vi "_BMarkInfo to MCTable.vi"(11 "BookmarkInfo":T1=[{"Bookmark ID"=1689, "Bookmark Tag"="#CSM", "Label Text"="#CSM State Syntax\n\n// Comment line, all text to the right of “//” will be ignored\n// Local Message Example\nDoSth: DoA >> Arguments\n\n// Sync Call Example\nAPI: xxxx >> Arguments -@ TargetModule\n\n// Async Call Example\nAPI: xxxx >> Arguments -> TargetModule\n\n// Async Call without Reply Example\nAPI: xxxx >> Arguments ->| TargetModule\n\n// Broadcast normal status:\nStatus >> StatusArguments  -><status>\n\n// Broadcast Interrupt status:\nInterrupt >> StatusArguments  -><interrupt>\n\n// Register Source Module's status to Handler Module\nStatus@Source Module >> Handler Module@Handler Module -><register>\n\n// Unegister Source Module's status\nStatus@Source Module >> Handler Module -><unregister>"}, {"Bookmark ID"=1690, "Bookmark Tag"="#CSM", "Label Text"="#CSM README FIRST\n\r\nCSM is a LabVIEW application framework that builds upon JKI State Machine (JKISM). It follows the pattern of JKISM and extends the keywords to describe message communication between CSM modules, including concepts such as Sync-Message, Async-Message, Subscription/Unsubscription of status - essential elements for creating reusable code modules. \n\nFor more information, please visit the CSM wiki: https://github.com/NEVSTOP-LAB/JKI-State-Machine-Plus-Plus/wiki\r\n\r\nFor instructions on JKI State Machine, visit: \n    http://jki.net/state-machine/\r\nFor information about CSM, visit: \n    https://github.com/NEVSTOP-LAB"}, {"Bookmark ID"=1850, "Bookmark Tag"="#CSM-Example", "Label Text"="#CSM-Example Step1"}, {"Bookmark ID"=1877, "Bookmark Tag"="#CSM-Example", "Label Text"="#CSM-Example Step4.2"}, {"Bookmark ID"=1879, "Bookmark Tag"="#CSM-Example", "Label Text"="#CSM-Example Step4.1"}, {"Bookmark ID"=1889, "Bookmark Tag"="#CSM-Example", "Label Text"="#CSM-Example Step5.1"}, {"Bookmark ID"=1907, "Bookmark Tag"="#CSM-Example", "Label Text"="#CSM-Example Step5.2"}, {"Bookmark ID"=1952, "Bookmark Tag"="#CSM-Example", "Label Text"="#CSM-Example Step5.3"}, {"Bookmark ID"=1955, "Bookmark Tag"="#CSM-Example", "Label Text"="#CSM-Example Step5.4"}, {"Bookmark ID"=1992, "Bookmark Tag"="#CSM-Example", "Label Text"="#CSM-Example Step5.5"}, {"Bookmark ID"=2001, "Bookmark Tag"="#CSM-Example", "Label Text"="#CSM-Example Step5.6"}, {"Bookmark ID"=2043, "Bookmark Tag"="#CSM-Example", "Label Text"="#CSM-Example Step5.7"}, {"Bookmark ID"=2087, "Bookmark Tag"="#CSM-Example", "Label Text"="#CSM-Example Step5.8"}, {"Bookmark ID"=2123, "Bookmark Tag"="#CSM-Example", "Label Text"="#CSM-Example Step5.8"}, {"Bookmark ID"=2353, "Bookmark Tag"="#CSM-Example", "Label Text"="#CSM-Example Step2.2"}, {"Bookmark ID"=2382, "Bookmark Tag"="#CSM-Example", "Label Text"="#CSM-Example Step2.1"}, {"Bookmark ID"=2400, "Bookmark Tag"="#CSM-Example", "Label Text"="#CSM-Example Step3"}, {"Bookmark ID"=2417, "Bookmark Tag"="#CSM-Example", "Label Text"="#CSM-Example Step6"}, {"Bookmark ID"=2477, "Bookmark Tag"="#CSM-Example", "Label Text"="#CSM-Example Step7"}, {"Bookmark ID"=2527, "Bookmark Tag"="#CSM-Example", "Label Text"="#CSM-Example Step8"}, {"Bookmark ID"=2547, "Bookmark Tag"="#CSM-Example", "Label Text"="#CSM-Example Step9"}, {"Bookmark ID"=2598, "Bookmark Tag"="#CSM-Example", "Label Text"="#CSM-Example Steps\r\rBased on JKISM, CSM includes the following major extended features:\r\r- Step 1: CSM is a program framework, so it requires a module name.\r- Step 2: CSM redesigns the core string parsing engine.\r  - Step 2.1: JKISM uses `Parse State Queue.vi`, which only outputs the next state queue and its corresponding arguments (located after `>>`), primarily functioning as a \"Dequeue Element\" operation.\r  - Step 2.2: CSM uses `Parse State Queue++.vi`, which adds the following major features:\r    - Automatically creates/handles/destroys the queue/user event mechanism based on the state queue input, so the user only needs to provide the corresponding high-level string messages.\r    - Enables Inter-module/Inter-VI message transmission.\r    - Includes additional inputs, such as Dequeue Timeout, Response Timeout, and Allowed Messages, to implement more advanced functionality.\r- Step 3: CSM adds an internal state debugging log, `history.vi`, for better debugging and recording. The state history can be displayed directly on the front panel.\r- Step 4: CSM defines a series of string syntaxes to implement local/inter-module message transmission, such as synchronous messages, asynchronous messages, state creation/registration/unregistration, etc.\r  - Step 4.1: JKISM only defines local state transitions. It can carry an argument and comment.\r  - Step 4.2: CSM is a software framework, so it defines modules and message communication between modules.\r- Step 5: CSM defines some base states to handle the logical behavior of communication between modules.\r  - Step 5.1: \"Critical Error\" is used to handle unrecoverable errors.\r  - Step 5.2: \"Target Timeout Error\" is used to handle module message communication timeout errors.\r  - Step 5.3: \"Target Error\" is used to handle errors where the target module does not exist.\r  - Step 5.4: \"Async Response\" is used to handle replies to asynchronous messages.\r  - Step 5.5: \"Response\" is used to handle replies to synchronous messages.\r  - Step 5.6: \"Async Message Posted\" is used to handle operations after an asynchronous message is sent.\r  - Step 5.7: (Optional) Message events used in \"Events: Register\" and \"Events: Unregister\" are used to trigger a CSM module with an event structure to exit the structure.\r  - Step 5.8: (Optional) `<New State Notifier Event>` works with Step 5.7 to break out of the event structure and wait when an external message arrives.\r  - Step 5.9: (Optional) CSM recommends using API groups to provide external interfaces, but in reality, all cases can be called using messages.\r- Step 6: CSM additionally defines \"Msg/Rsp's CSM\" to locate the source module of external messages and states.\r- Step 7: Additional message information, such as the source message name and source arguments of a response, can be obtained here.\r- Step 8: CSM has preset message returns.\r- Step 9: CSM extends debugging tools. For details, please refer to the palette CSM -> CSM Debug Tools."}, {"Bookmark ID"=2599, "Bookmark Tag"="#CSM-Example", "Label Text"="#CSM-Example Introduction\r\rThis example compares the code between the JKISM framework and the CSM framework. Both frameworks use string-based message queues to implement the core state machine.\r"}]) -> (3 "sorted 2D array":string[][](array[string])=[["#CSM-Example Step1", "1850", "#CSM-Example"], ["#CSM-Example Step4.2", "1877", "#CSM-Example"], ["#CSM-Example Step4.1", "1879", "#CSM-Example"], ["#CSM-Example Step5.1", "1889", "#CSM-Example"], ["#CSM-Example Step5.2", "1907", "#CSM-Example"], ["#CSM-Example Step5.3", "1952", "#CSM-Example"], ["#CSM-Example Step5.4", "1955", "#CSM-Example"], ["#CSM-Example Step5.5", "1992", "#CSM-Example"], ["#CSM-Example Step5.6", "2001", "#CSM-Example"], ["#CSM-Example Step5.7", "2043", "#CSM-Example"], ["#CSM-Example Step5.8", "2087", "#CSM-Example"], ["#CSM-Example Step5.8", "2123", "#CSM-Example"], ["#CSM-Example Step2.2", "2353", "#CSM-Example"], ["#CSM-Example Step2.1", "2382", "#CSM-Example"], ["#CSM-Example Step3", "2400", "#CSM-Example"], ["#CSM-Example Step6", "2417", "#CSM-Example"], ["#CSM-Example Step7", "2477", "#CSM-Example"], ["#CSM-Example Step8", "2527", "#CSM-Example"], ["#CSM-Example Step9", "2547", "#CSM-Example"], ["#CSM-Example Steps", "2598", "#CSM-Example"], ["#CSM-Example Introduction", "2599", "#CSM-Example"]])   [LabVIEW 2017, in "CSM_ExampleBrowser.lvlib"]
uses:
  CSM_ExampleBrowser.lvlib
  <vilib>/Utility/miscctls.llb/LVBookmarkInfoTypeDef.ctl
  Communicable State Machine.lvlib
  _Shared/CSM Shared.lvlib
panel:
  out "sorted array":dbl[](array[numeric])
  out "Array 4":cluster{string[]}[](array[cluster])
  out "Array 3":string[](array[string])=["#CSM-Example Introduction", "#CSM-Example Step", "#CSM-Example Steps"]
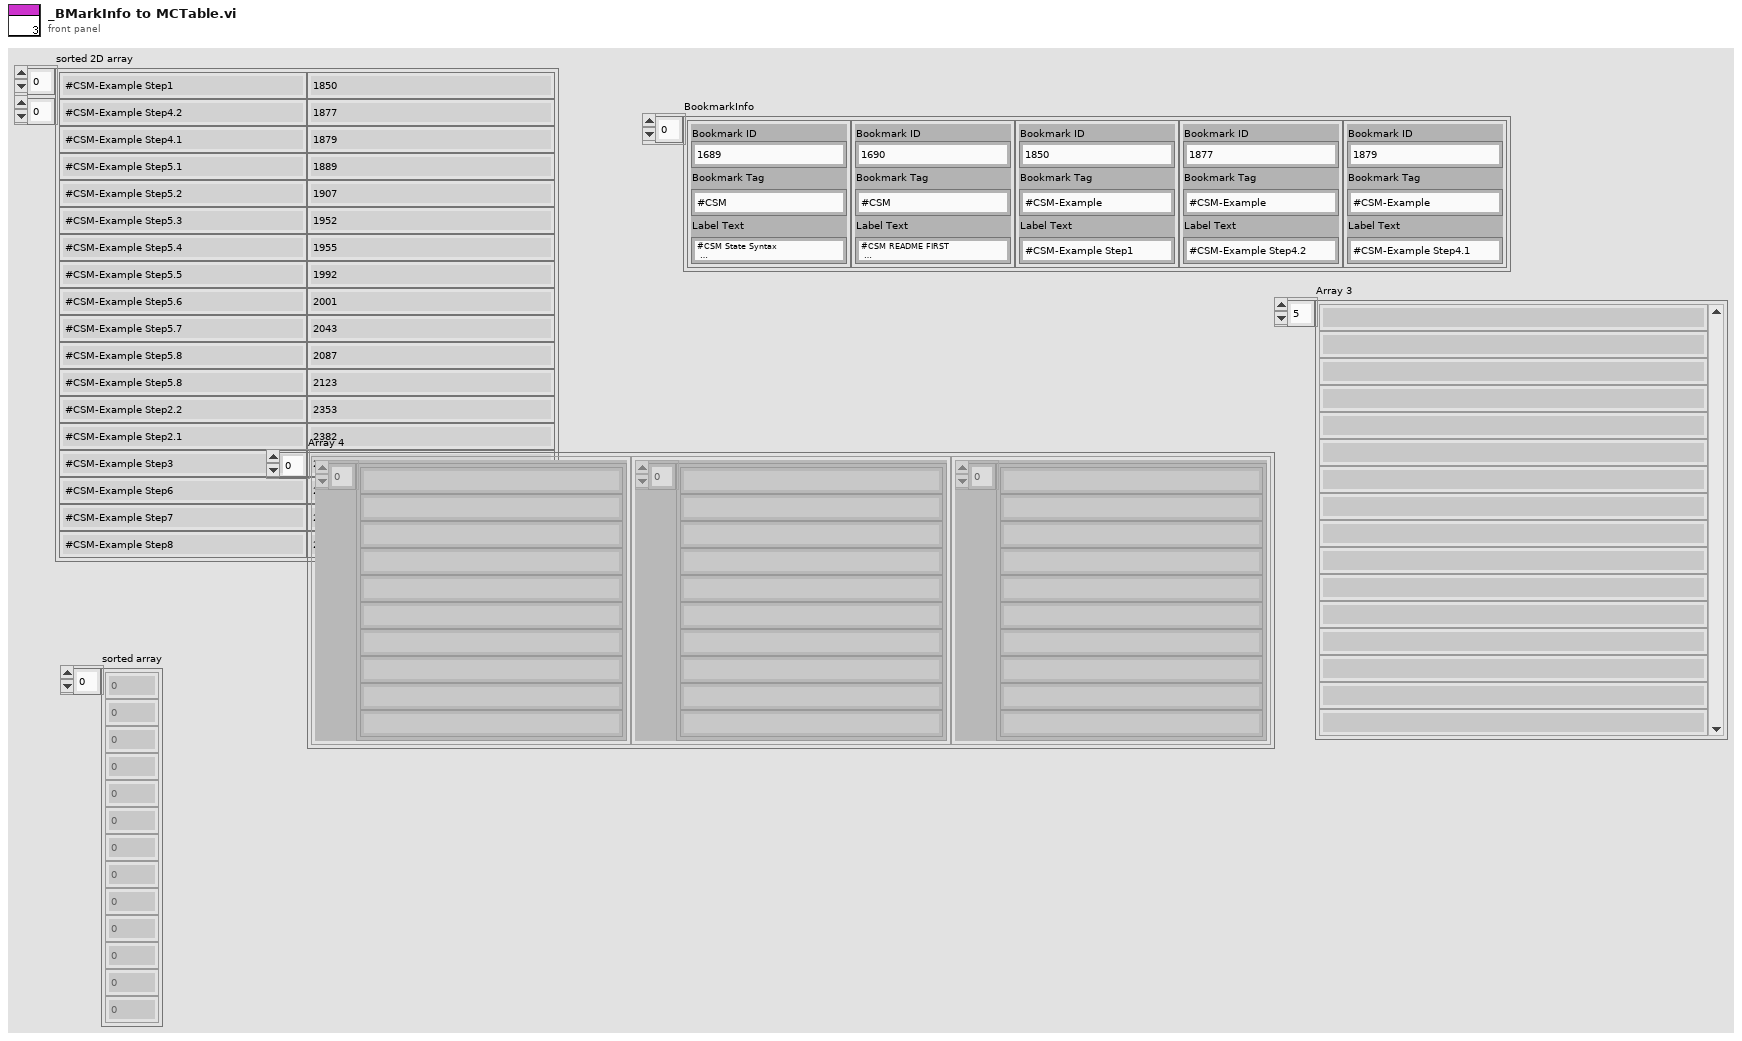
[diagram p1: front panel]
types:
  T1 = typedef "LVBookmarkInfoTypeDef.ctl" = cluster{"Bookmark ID":u32, "Bookmark Tag":string, "Label Text":string}[]
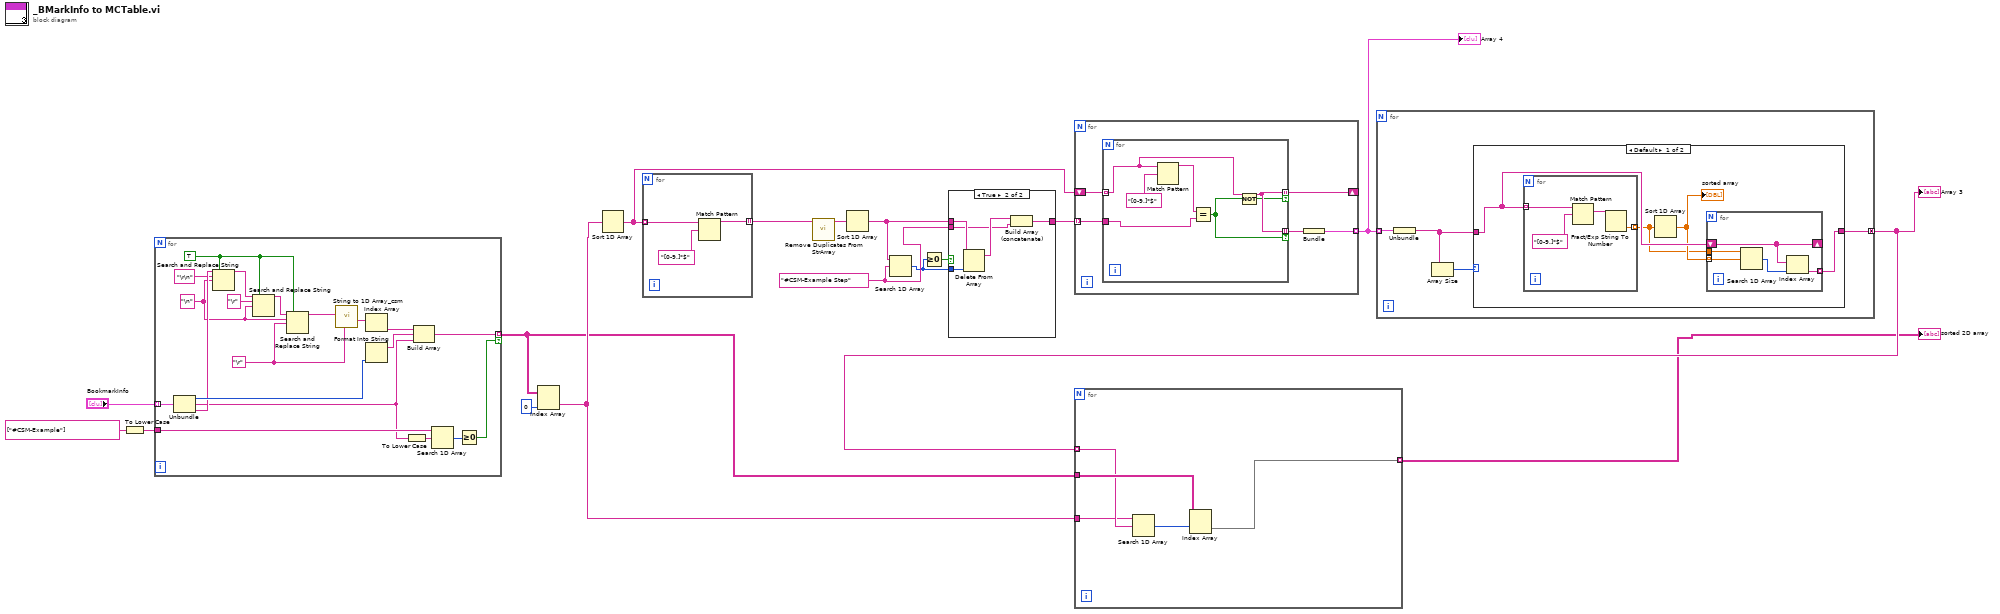
[diagram p0: block diagram]
diagram:
  w4 = "#CSM-Example Step" ("element")
  n1 = To Lower Case(string=string[] ["#CSM-Example"]) -> (all lower case string=w15:string[])
  n2 = for {
    tunnel: "BookmarkInfo" -> [w37] mode=indexing
    tunnel: [w34] -> w7 mode=indexing if=w18
    tunnel: w15 -> [w23]
    w28 = TRUE ("replace all? (F)")
    w30 = "\n" ("search string")
    w24 = "\r"
    n3 = Unbundle(w37) -> ("Bookmark ID"=w36:u32, "Bookmark Tag"=w22:string, "Label Text"=w33:string)
    n4 = Search and Replace String(replace all?=w28, input string=w33, search string="\r\n", replace string=w30) -> (result string=w25:string)  [unwired: 4 in, 3 out]
    n5 = Search and Replace String(replace all?=w28, input string=w25, search string="\r", replace string=w30) -> (result string=w27:string)  [unwired: 4 in, 3 out]
    n6 = Search and Replace String(replace all?=w28, input string=w27, search string=w30, replace string=w24) -> (result string=w31:string)  [unwired: 4 in, 3 out]
    n7 = call "String to 1D Array_csm.vi"("delimiter (Tab)"=w24, "string"=w31) -> ("Array of Strings"=w32:string[])  [unwired: 9 in]
    n8 = Index Array(array=w32) -> (element=w19:string)  [unwired: 1 in]
    n9 = Format Into String(w36) -> (resulting string=w35:string)  [unwired: 3 in, 1 out]
    n10 = To Lower Case(string=w22) -> (all lower case string=w21:string)
    n11 = Build Array(w19, w35, w22) -> (w34:string[])
    n12 = Search 1D Array(1D array=w23, element=w21) -> (index of element=w20:i32)  [unwired: 1 in]
    n13 = Greater Or Equal To 0?(x=w20) -> (x >= 0?=w18:bool)
  }
  n14 = Index Array(array=w7, index (col)=0 ("disabled index (col)")) -> (element=w8:string[])  [unwired: 1 in]
  n15 = Sort 1D Array(array=w8) -> (sorted array=w12:string[])
  n16 = for {
    tunnel: w12 -> [w40] mode=indexing
    tunnel: [w38] -> w14 mode=indexing
    n17 = Match Pattern(string=w40, regular expression="[0-9.]*$") -> (before substring=w38:string)  [unwired: 1 in, 3 out]
  }
  n18 = call "Remove Duplicates From StrArray.vi"("StrArray In"=w14) -> ("StrArray"=w13:string[])  [unwired: 9 in, 1 out]
  n19 = Sort 1D Array(array=w13) -> (sorted array=w3:string[])
  n20 = Search 1D Array(1D array=w3, element=w4) -> (index of element=w1:i32)  [unwired: 1 in]
  n21 = Greater Or Equal To 0?(x=w1) -> (x >= 0?=w2:bool)
  n22 = case shown="True" w2 {
    tunnel: w1 -> [_ w46]
    tunnel: [w41 w45] -> w5
    tunnel: w4 -> [_ w42]
    tunnel: w3 -> [w41 w44]
    frame False {
    }
    frame True {
      n23 = Delete From Array(array=w44, index=w46) -> (array with subset deleted=w43:string[])  [unwired: 1 in, 1 out]
      n24 = Build Array (concatenate)(w43, w42) -> (w45:string[])
    }
  }
  n25 = for {
    tunnel: w5 -> [w51] mode=indexing
    shift-right: [w47] -> _
    shift-left: w12 -> [w50]
    tunnel: [w48] -> w11 mode=indexing
    n26 = for {
      tunnel: w51 -> [w56]
      tunnel: w50 -> [w53] mode=indexing
      tunnel: [w53] -> w47 mode=indexing if=w52
      tunnel: [w53] -> w49 mode=indexing if=w57
      n27 = Match Pattern(string=w53, regular expression="[0-9.]*$") -> (before substring=w54:string)  [unwired: 1 in, 3 out]
      n28 = Equal?(x=w54, y=w56) -> (x = y?=w57:bool)
      n29 = Not(x=w57) -> (.not. x?=w52:bool)
    }
    n30 = Bundle(w49) -> (w48:cluster{string[]})  [unwired: 1 in]
  }
  "Array 4" <- w11
  n31 = for {
    tunnel: w11 -> [w61] mode=indexing
    tunnel: [w59] -> w9 mode=concatenating
    n32 = Unbundle(w61) -> (w58:string[])
    n33 = Array Size(array=w58) -> (size(s)=w60:i32)
    n34 = case shown="Default" w60 {
      tunnel: [w62 w75] -> w59
      tunnel: w58 -> [w65 w75]
      frame Default {
        n35 = for {
          tunnel: w65 -> [w74] mode=indexing
          tunnel: [w71] -> w63 mode=indexing
          n36 = Match Pattern(string=w74, regular expression="[0-9.]*$") -> (match substring=w72:string)  [unwired: 1 in, 3 out]
          n37 = Fract/Exp String To Number(string=w72) -> (number=w71:dbl)  [unwired: 3 in, 1 out]
        }
        n38 = Sort 1D Array(array=w63) -> (sorted array=w64:dbl[])
        "sorted array" <- w64
        n39 = for {
          shift-right: [w67] -> _
          shift-left: w65 -> [w67]
          tunnel: w64 -> [w70] mode=indexing
          tunnel: w63 -> [w69]
          tunnel: [w66] -> w62 mode=indexing
          n40 = Search 1D Array(1D array=w69, element=w70) -> (index of element=w68:i32)  [unwired: 1 in]
          n41 = Index Array(array=w67, index=w68) -> (element=w66:string)
        }
      }
      frame 0, 1 {
      }
    }
  }
  "Array 3" <- w9
  n42 = for {
    tunnel: w7 -> [w80]
    tunnel: w9 -> [w79] mode=indexing
    tunnel: w8 -> [w78]
    tunnel: [w76] -> w6 mode=indexing
    n43 = Search 1D Array(1D array=w78, element=w79) -> (index of element=w77:i32)  [unwired: 1 in]
    n44 = Index Array(array=w80, index (row)=w77) -> (element=w76:string[])  [unwired: 1 in]
  }
  "sorted 2D array" <- w6
